vi "1 Angle to Rotational Velocity.vi"(1 "Robot\nHeading":T2 format="%05.1f") -> (0 "Robot\nRate of Turn":T1 format="%05.1f")   [LabVIEW 2011]
doc: "uses the low-pass differentiator to estimate velocity from a series of robot locations.\nTODO: does not deal with switches between UTM zones."
uses:
  2 Typedefs/heading.ctl
  2 Typedefs/rate of turn.ctl
  Low Pass Differentiator - Heading.vi
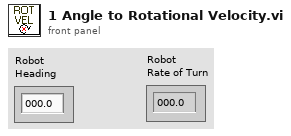
[diagram p1: front panel]
types:
  T1 = typedef "rate of turn.ctl" = dbl
  T2 = typedef "heading.ctl" = dbl
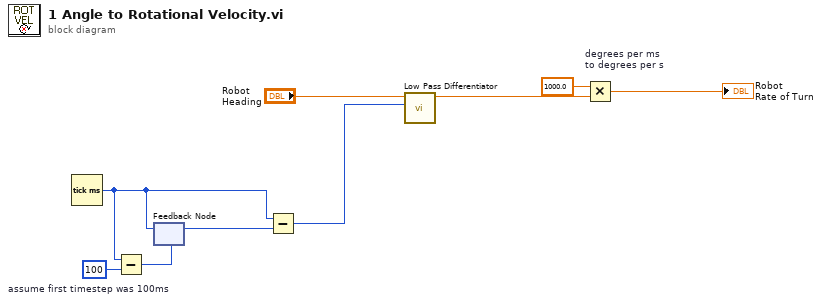
[diagram p0: block diagram]
diagram:
  w8 = u32 100  # assume first timestep was 100ms
  n1 = Tick Count (ms)() -> (millisecond timer value=w7:u32)
  n2 = Subtract(x=w7, y=w8) -> (x-y=w6:u32)
  n3 = feedback #1(w6) -> (w5:u32)
  n4 = feedback-in #1(w7) -> ()
  n5 = Subtract(x=w7, y=w5) -> (x-y=w9:u32)
  n6 = call-poly "Low Pass Differentiator.vi"("dt"=w9, "Heading"="Robot\nHeading") -> ("Heading Change, smoothed"=w4:dbl)  [unwired: 9 in]
  n7 = Multiply "degrees per ms\nto degrees per s"(x=1000.0, y=w4) -> (x*y=→"Robot\nRate of Turn":dbl)
